vi "Panel.vi"(11 "Panel In":refnum<class "DeviceDetailPanel.lvclass">) -> ()   [LabVIEW 2020, in "PicoG-App.lvlib" / "DeviceDetailPanel.lvclass"]
uses:
  DeviceDetailPanel.lvclass
  C:/Program Files (x86)/National Instruments/LabVIEW 2020/vi.lib/IlluminatedG/IG OOPanel/OOPanel/Panel/Panel.lvclass
  <vilib>/IlluminatedG/IG OOPanel/OOPanel/Panel/Basic UI State.ctl
  Terminal State.ctl
  DeviceDetailPanel.lvclass/DeviceDetailPanel.ctl
  ViaApp/ViaApp.lvclass
  Device/Device.lvclass
  Builds/picoG/ppl/PicoG-Core.lvlibp/PicoG-Processor/PicoG-Core/Platform/Platform.lvclass
  <vilib>/IlluminatedG/IG OOPanel/OOPanel/Panel/Panel.lvclass
  <vilib>/IlluminatedG/IG OOPanel/OOPanel/OOPanel.lvlib
panel:
  out "Picture":picture
  in  "Remove":bool
  out "Alias":string
  in  "Set Alias":bool
  out "Version":string
  out "Board":string
  out "Platform":string
  out "ID":string
  out "Device Status":string="Unknown"
  out "Terminal Status":string
  in  "Close":bool
  in  "Open":bool
  out "Terminal":string
  # "Platform"
  # "Board"
  # "Serial"
  # "Version"
  # "Status"
  # "Terminal"
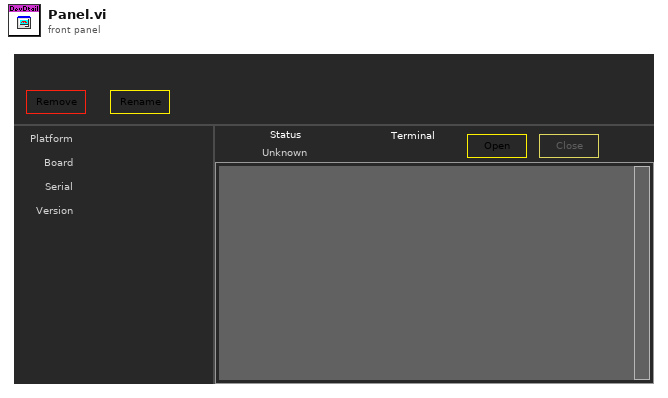
[diagram p1: front panel]
types:
  T1 = typedef "OOPanel.lvlib/Panel.lvclass/Basic UI State.ctl" = enum16{"Init", "Run", "Close"}
  T2 = typedef "PicoG-App.lvlib/DeviceDetailPanel.lvclass/Terminal State.ctl" = enum16{"Disconnected", "Connecting", "Connected", "Error"}
  T3 = enum8{"Enabled", "Disabled", "Disabled and Grayed Out"}
  T4 = typedef "PicoG-App.lvlib/DeviceDetailPanel.lvclass/Inbound Events.ctl" = cluster{"Device Updated":refnum<user-event>, "Deploy":refnum<user-event>}
  T5 = typedef "OOPanel.lvlib/Panel.lvclass/Panel Events.ctl" = cluster{"Visbility":refnum<user-event>, "Close":refnum<user-event>}
  T6 = typedef "PicoG-App.lvlib/DeviceDetailPanel.lvclass/Ref Data.ctl" = cluster{"Device":refnum<class "Device.lvclass">}
  T7 = typedef "OOPanel.lvlib/Panel.lvclass/Visibility State.ctl" = enum16{"Idle", "Closed", "Hidden", "Visible", "Subpanel"}
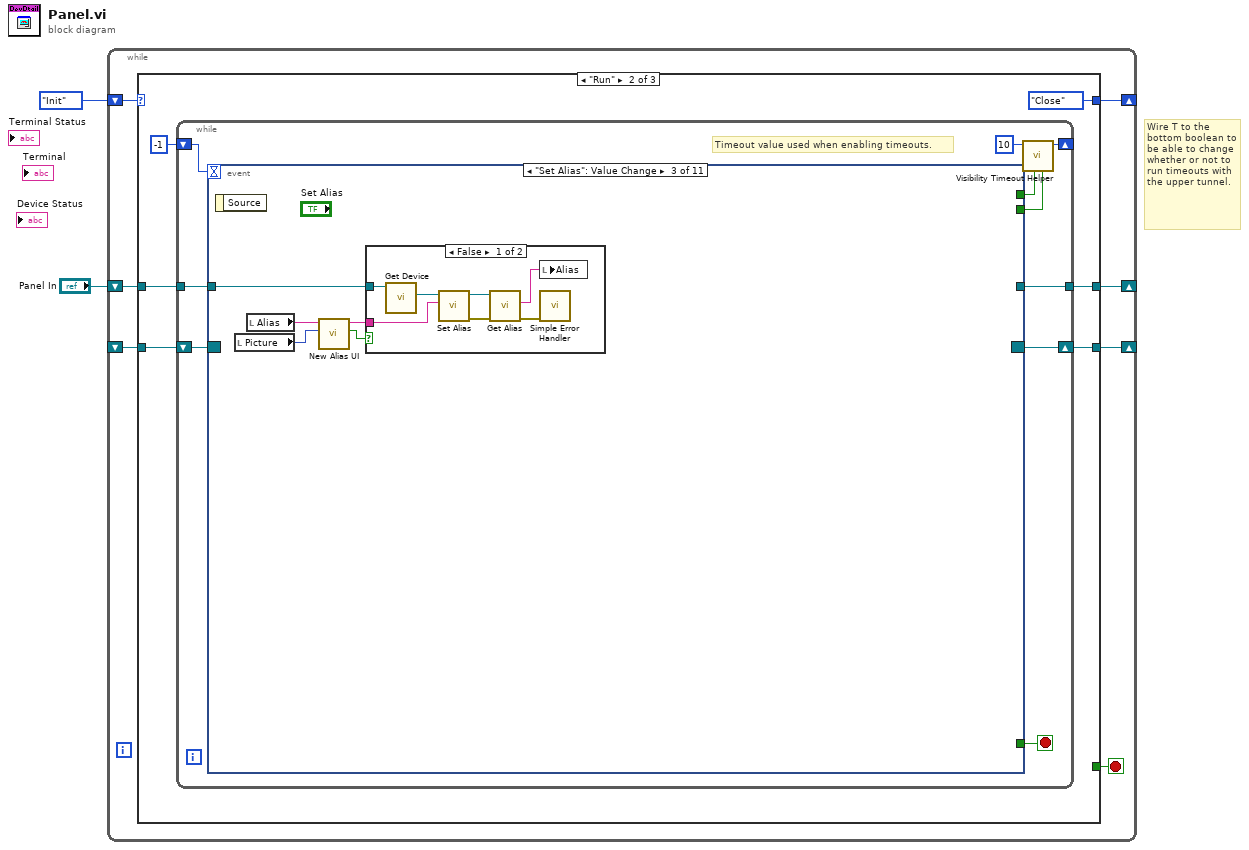
[diagram p0: block diagram]
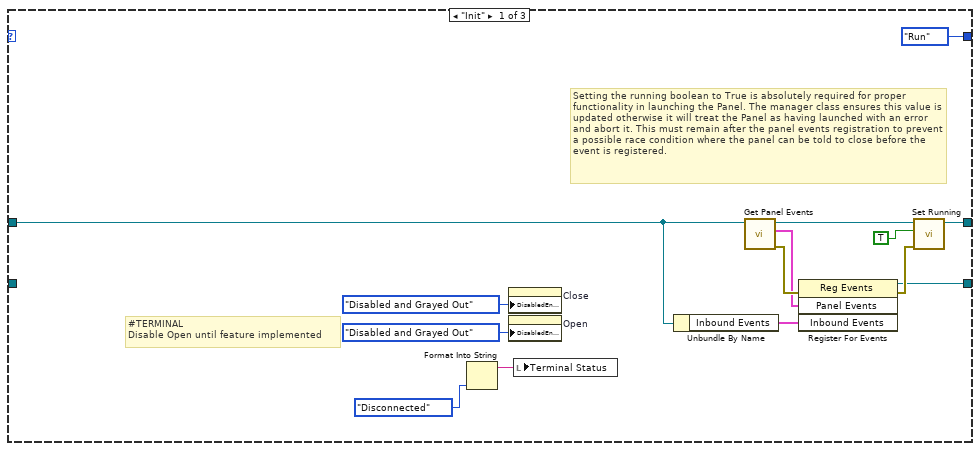
[diagram p2: hidden frame]
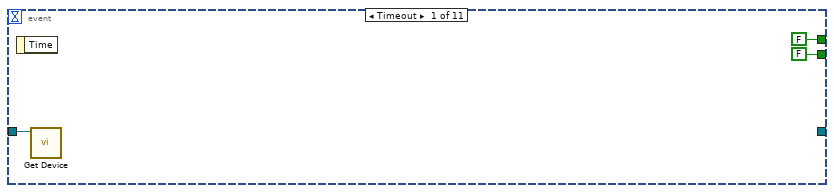
[diagram p3: hidden frame]
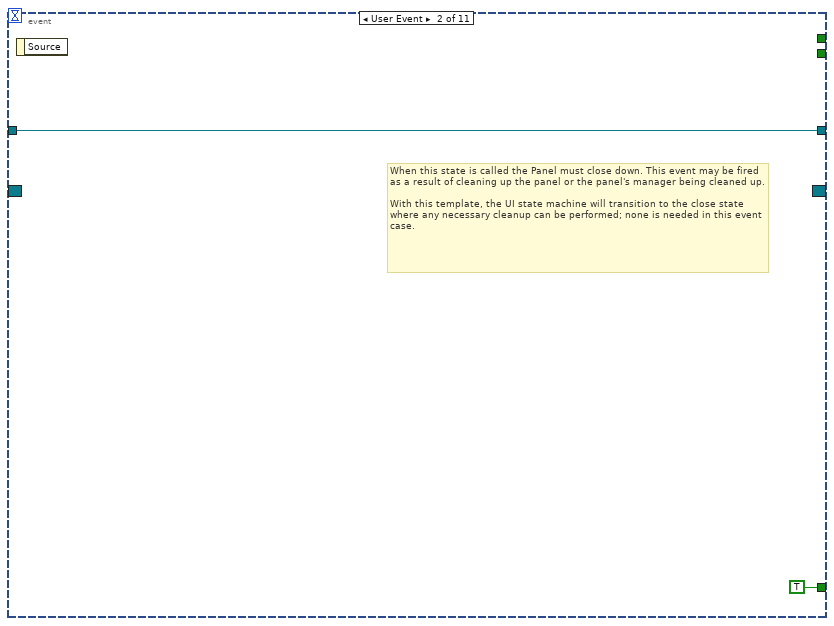
[diagram p4: hidden frame]
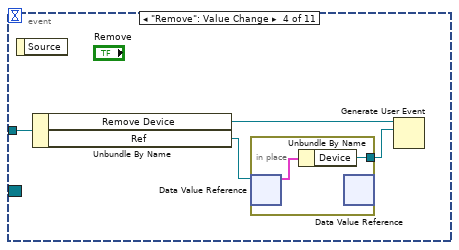
[diagram p6: hidden frame]
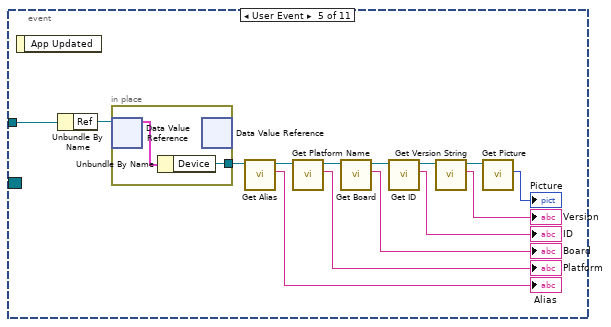
[diagram p7: hidden frame]
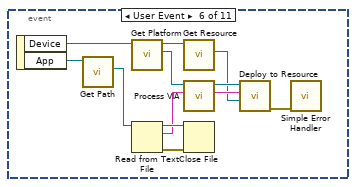
[diagram p8: hidden frame]
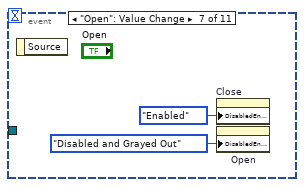
[diagram p9: hidden frame]
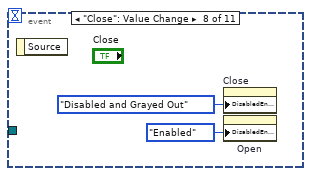
[diagram p10: hidden frame]
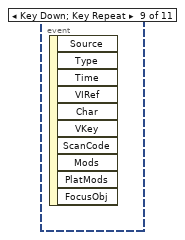
[diagram p11: hidden frame]
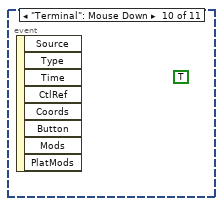
[diagram p12: hidden frame]
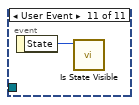
[diagram p13: hidden frame]
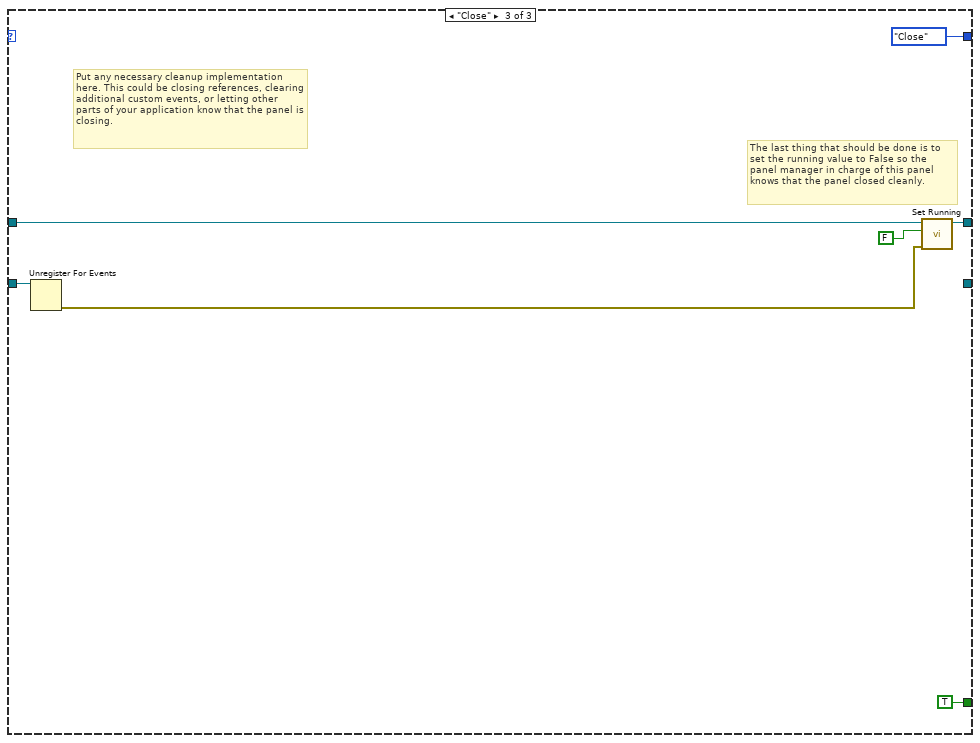
[diagram p14: hidden frame]
diagram:
  # "Wire T to the bottom boolean to be able to change whether or not to run timeouts with the upper tunnel."
  n1 = while {
    shift-right: [w8] -> _
    shift-left: _ -> [w9]
    shift-right: [w6] -> _
    shift-left: Basic_UI_State."Init" ("Basic UI State") -> [w7]
    shift-right: [w4] -> _
    shift-left: "Panel In" -> [w3]
    stop <- w5 stop-if-true
    n2 = case shown="\"Run\"" w7 {
      tunnel: w9 -> [_ w29 w98]
      tunnel: [w17 w27 _] -> w8
      tunnel: [Basic_UI_State."Run" ("Basic UI State") Basic_UI_State."Close" ("Basic UI State") Basic_UI_State."Close" ("Basic UI State")] -> w6
      tunnel: [_ _ TRUE] -> w5
      tunnel: [w16 w24 w96] -> w4
      tunnel: w3 -> [w11 w25 w97]
      frame "Init" {
        # "#TERMINAL\nDisable Open until feature implemented"
        # "Setting the running boolean to True is absolutely required for proper functionality in launching the Panel. The manager class ensures this value is updated otherwise it will treat the Panel as having launched with an error and abort it. This must remain after the panel events registration to prevent a possible race condition where the panel can be told to close before the event is registered."
        n3 = Format Into String(Terminal_State."Disconnected" ("Terminal State")) -> (resulting string=w13:string)  [unwired: 3 in, 1 out]
        n4 = property on="Close" class="Bool"("DisabledEnum"=T3."Disabled and Grayed Out" ("Disabled")) -> ()  [unwired: 2 in, 2 out]
        n5 = property on="Open" class="Bool"("DisabledEnum"=T3."Disabled and Grayed Out" ("Disabled")) -> ()  [unwired: 2 in, 2 out]
        n6 = local write "Terminal Status"(w13) -> ()
        n7 = Unbundle By Name(w11) -> ("Inbound Events"=w10:T4)
        n8 = call <vilib>:"Get Panel Events.vi"("Panel in"=w11) -> ("error out"=w23:errorcluster, "Panel Events"=w19:T5, "Panel out"=w20:refnum<class "DeviceDetailPanel.lvclass">)  [unwired: 8 in]
        n9 = register-events(error in=w23, w19, w10) -> (reference out=w17:refnum<event-registration>, error out=w21:errorcluster)  [unwired: 1 in]
        n10 = call <vilib>:"Set Running.vi"("error in (no error)"=w21, "Running"=TRUE, "Panel in"=w20) -> ("Panel out"=w16:refnum<class "DeviceDetailPanel.lvclass">)  [unwired: 7 in, 1 out]
      }
      frame "Run" {
        n11 = while {
          shift-right: [w35] -> w27
          shift-left: w29 -> [w36]
          shift-right: [w38] -> _
          shift-left: -1 ("Timeout") -> [w37]
          tunnel: w25 -> [w31]
          tunnel: [w30] -> w24
          stop <- w32 stop-if-true
          # "Timeout value used when enabling timeouts."
          n12 = event shown="[2] \"Set Alias\": Value Change" {
            selector: w36 -> [_ _ _ _ _ _ _ _ _ _ _]
            dyn-events: [_ _ _ _ _ _ _ _ _ _ _] -> w35
            timeout: w37 -> [_ _ _ _ _ _ _ _ _ _ _]
            tunnel: [FALSE _ _ _ _ _ _ _ _ _ _] -> w34
            tunnel: [FALSE _ _ _ _ _ _ _ _ _ _] -> w33
            tunnel: [_ TRUE _ _ _ _ _ _ _ _ _] -> w32
            tunnel: w31 -> [w40 w43 w46 w59 w75 _ _ _ _ _ _]
            tunnel: [_ w43 _ _ _ _ _ _ _ _ _] -> w30
            event Timeout {
              n13 = event-data() -> ()  [unwired: 1 in, 1 out]
              n14 = call "Get Device.vi"("DeviceDetailPanel in"=w40) -> ()  [unwired: 8 in, 3 out]
            }
            event User Event {
              # "When this state is called the Panel must close down. This event may be fired as a result of cleaning up the panel or the panel's manager being cleaned up.\n\nWith this template, the UI state machine will transition to the close state where any necessary cleanup can be performed; none is needed in this event case."
              n15 = event-data() -> ()  [unwired: 1 in, 1 out]
            }
            event "Set Alias": Value Change {
              n16 = event-data() -> ()  [unwired: 1 in, 1 out]
              n17 = local read "Picture"() -> (w45:picture)
              n18 = local read "Alias"() -> (w48:string)
              n19 = call "New Alias UI.vi"("Picture"=w45, "Current Alias"=w48) -> ("Cancelled"=w49:bool, "Alias"=w47:string)  [unwired: 8 in]
              n20 = case shown="False" w49 {
                tunnel: w47 -> [w54 _]
                tunnel: w46 -> [w56 _]
                frame False {
                  n21 = call "Get Device.vi"("DeviceDetailPanel in"=w56) -> ("Device"=w55:refnum<class "Device.lvclass">)  [unwired: 8 in, 2 out]
                  n22 = call "Set Alias.vi"("Alias"=w54, "Device in"=w55) -> ("error out"=w52:errorcluster, "Device out"=w53:refnum<class "Device.lvclass">)  [unwired: 8 in]
                  n23 = call "Get Alias.vi"("error in (no error)"=w52, "Device in"=w53) -> ("error out"=w50:errorcluster, "Alias"=w51:string)  [unwired: 7 in, 1 out]
                  n24 = local write "Alias"(w51) -> ()
                  n25 = call <vilib>:"Simple Error Handler.vi"("error in (no error)"=w50) -> ()  [unwired: 4 in, 5 out]
                }
                frame True {
                }
              }
            }
            event "Remove": Value Change {
              n26 = event-data() -> ()  [unwired: 1 in, 1 out]
              n27 = Unbundle By Name(w59) -> ("Remove Device"=w58:refnum<user-event>, "Ref"=w60:refnum<data-value>)
              n28 = in-place {
                in-place-border: [w61] -> w57
                n29 = in-place-dvr #1(w60) -> (w62:T6)  [unwired: 1 out]
                n30 = Unbundle By Name(w62) -> ("Device"=w61:refnum<class "Device.lvclass">)
                n31 = in-place-dvr #1() -> ()  [unwired: 1 in, 2 out]
              }
              n32 = Generate User Event(user event=w58, event data cluster=w57) -> ()  [unwired: 2 in, 2 out]
            }
            event User Event {
              n33 = event-data() -> ()  [unwired: 1 in, 1 out]
              n34 = Unbundle By Name(w75) -> ("Ref"=w76:refnum<data-value>)
              n35 = in-place {
                in-place-border: [w77] -> w74
                n36 = in-place-dvr #2(w76) -> (w78:T6)  [unwired: 1 out]
                n37 = Unbundle By Name(w78) -> ("Device"=w77:refnum<class "Device.lvclass">)
                n38 = in-place-dvr #2() -> ()  [unwired: 1 in, 2 out]
              }
              n39 = call "Get Alias.vi"("Device in"=w74) -> ("Alias"=→"Alias":string, "Device out"=w72:refnum<class "Device.lvclass">)  [unwired: 8 in, 1 out]
              n40 = call "Get Platform Name.vi"("Device in"=w72) -> ("Platform"=→"Platform":string, "Device out"=w70:refnum<class "Device.lvclass">)  [unwired: 8 in, 1 out]
              n41 = call "Get Board.vi"("Device in"=w70) -> ("Board"=→"Board":string, "Device out"=w68:refnum<class "Device.lvclass">)  [unwired: 8 in, 1 out]
              n42 = call "Get ID.vi"("Device in"=w68) -> ("Id"=→"ID":string, "Device out"=w66:refnum<class "Device.lvclass">)  [unwired: 8 in, 1 out]
              n43 = call "Get Version String.vi"("Device in"=w66) -> ("Version"=→"Version":string, "Device out"=w64:refnum<class "Device.lvclass">)  [unwired: 8 in, 1 out]
              n44 = call "Get Picture.vi"("Device in"=w64) -> ("Picture"=→"Picture":picture)  [unwired: 8 in, 2 out]
            }
            event User Event {
              n45 = event-data() -> ("Device"=w90:refnum<class "Device.lvclass">, "App"=w81:refnum<class "ViaApp.lvclass">)  [unwired: 1 in]
              n46 = call "Get Path.vi"("ViaApp in"=w81) -> ("Path"=w79:path)  [unwired: 8 in, 2 out]
              n47 = call "Get Platform.vi"("Device in"=w90) -> ("Platform"=w88:refnum<class "Platform.lvclass">, "Device out"=w89:refnum<class "Device.lvclass">)  [unwired: 8 in, 1 out]
              n48 = Read from Text File(file (use dialog)=w79) -> (refnum out=w83:refnum<file>, text=w80:string, error out=w82:errorcluster)  [unwired: 3 in, 1 out]
              n49 = call "Get Resource.vi"("Device in"=w89) -> ("Resource"=w85:refnum<class "Resource.lvclass">)  [unwired: 8 in, 2 out]
              n50 = call-dynamic "Process VIA.vi"("Raw VIA"=w80, "DeployTarget in"=w88) -> ("VIA"=w86:string, "DeployTarget out"=w87:refnum<class "Platform.lvclass">)  [unwired: 7 in, 1 out]
              n51 = Close File(refnum=w83, error in=w82) -> ()  [unwired: 2 out]
              n52 = call-dynamic "Deploy to Resource.vi"("Resource"=w85, "VIA"=w86, "DeployTarget in"=w87) -> ("error out"=w84:errorcluster)  [unwired: 6 in, 2 out]
              n53 = call <vilib>:"Simple Error Handler.vi"("error in (no error)"=w84) -> ()  [unwired: 4 in, 5 out]
            }
            event "Open": Value Change {
              n54 = event-data() -> ()  [unwired: 1 in, 1 out]
              n55 = property on="Close" class="Bool"("DisabledEnum"=T3."Enabled" ("Disabled")) -> ()  [unwired: 2 in, 2 out]
              n56 = property on="Open" class="Bool"("DisabledEnum"=T3."Disabled and Grayed Out" ("Disabled")) -> ()  [unwired: 2 in, 2 out]
            }
            event "Close": Value Change {
              n57 = event-data() -> ()  [unwired: 1 in, 1 out]
              n58 = property on="Close" class="Bool"("DisabledEnum"=T3."Disabled and Grayed Out" ("Disabled")) -> ()  [unwired: 2 in, 2 out]
              n59 = property on="Open" class="Bool"("DisabledEnum"=T3."Enabled" ("Disabled")) -> ()  [unwired: 2 in, 2 out]
            }
            event Key Down; Key Repeat {
              n60 = event-data() -> ()  [unwired: 1 in, 10 out]
            }
            event "Terminal": Mouse Down {
              (unwired) TRUE ("Terminal Focused")
              n61 = event-data() -> ()  [unwired: 1 in, 8 out]
            }
            event User Event {
              n62 = event-data() -> ("State"=w95:T7)  [unwired: 1 in]
              n63 = call <vilib>:"Is State Visible.vi"("Visibility"=w95) -> ()  [unwired: 10 in, 1 out]
            }
          }
          n64 = call <vilib>:"Visibility Timeout Helper.vi"("Update?"=w33, "Use Timeout?"=w34, "Visible Timeout mS"=10) -> ("Timeout"=w38:i32)  [unwired: 8 in]
        }
      }
      frame "Close" {
        # "Put any necessary cleanup implementation here. This could be closing references, clearing additional custom events, or letting other parts of your application know that the panel is closing."
        # "The last thing that should be done is to set the running value to False so the panel manager in charge of this panel knows that the panel closed cleanly."
        n65 = Unregister For Events(event registration refnum=w98) -> (error out=w100:errorcluster)  [unwired: 1 in]
        n66 = call <vilib>:"Set Running.vi"("error in (no error)"=w100, "Running"=FALSE, "Panel in"=w97) -> ("Panel out"=w96:refnum<class "DeviceDetailPanel.lvclass">)  [unwired: 7 in, 1 out]
      }
    }
  }
